vi "RectRegionConstraint_New.vi"(9 "Constraint Data Cluster":variant, 10 "TopRightPoint":T1 {"Y" format="%14.3f"; "X" format="%14.3f"}, 11 "BottomLeftPoint":T1 {"Y" format="%14.3f"; "X" format="%14.3f"}) -> (3 "RECT_REGION_CONSTRAINT":T2={"BottomLeftPoint"={"X"=0.0, "Y"=0.0}, "TopRightPoint"={"X"=0.0, "Y"=0.0}, "Constraint"=variant, "Constraint Type"=enum."DIFF DRIVE KINEMATICS"} {"TopRightPoint"."Y" format="%14.3f"; "TopRightPoint"."X" format="%14.3f"; "BottomLeftPoint"."Y" format="%14.3f"; "BottomLeftPoint"."X" format="%14.3f"})   [LabVIEW 2019, in "Trajectory_Library.lvlib"]
doc: "Constructs a differential drive dynamics constraint.\n\n\nParameters:\n - MaxSpeed - Max speed (meters/sec)\n - DiffDriveKinematics - Diff Drive Kinematics data structure\n\nReturns\n - DiffDriveKineConstraint - Constraint data structure."
uses:
  Trajectory_Library.lvlib
  TRANSLATION2D.ctl
  TypeDef/TRAJ_CONSTRAINT_RECT_REGION.ctl
  Enum/TRAJ_CONSTRAINT_TYPES_ENUM.ctl
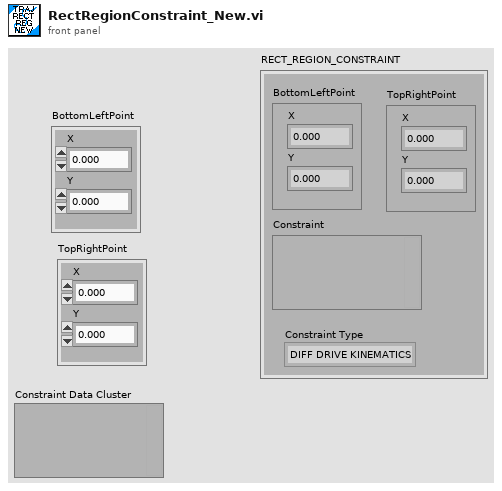
[diagram p1: front panel]
types:
  T1 = typedef "Trajectory_Library.lvlib/TRANSLATION2D.ctl" = cluster{"X":dbl, "Y":dbl}
  T2 = typedef "Trajectory_Library.lvlib/TRAJ_CONSTRAINT_RECT_REGION.ctl" = cluster{"BottomLeftPoint":T1, "TopRightPoint":T1, "Constraint":variant, "Constraint Type":T3}
  T3 = typedef "Trajectory_Library.lvlib/TRAJ_CONSTRAINT_TYPES_ENUM.ctl" = enum16{"UNDEFINED", "DIFF DRIVE KINEMATICS", "DIFF DRIVE VOLTAGE", "CENTRIPITAL ACCEL", "MECA DRIVE KINEMATICS", "SWERVE DRIVE KINEMATICS", "MAXIMUM VELOCITY"}
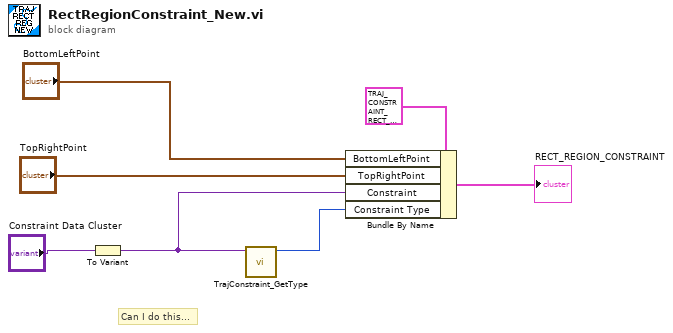
[diagram p0: block diagram]
diagram:
  # "Can I do this..."
  n1 = To Variant(anything="Constraint Data Cluster") -> (Variant=w2:variant)
  n2 = call "TrajConstraint_GetType.vi"("Trajectory Constraint"=w2) -> ("Trajectory Constraint Type"=w1:T3)  [unwired: 9 in, 1 out]
  n3 = Bundle By Name(cluster=T2 {"BottomLeftPoint"={"X"=0.0, "Y"=0.0}, "TopRightPoint"={"X"=0.0, "Y"=0.0}, "Constraint"=variant, "Constraint Type"=enum."DIFF DRIVE KINEMATICS"} ("RECT_REGION_CONSTRAINT"), "BottomLeftPoint"="BottomLeftPoint", "TopRightPoint"="TopRightPoint", "Constraint"=w2, "Constraint Type"=w1) -> (→"RECT_REGION_CONSTRAINT":T2)
